vi "Close DVRs.vi"(8 "error in (no error)":errorcluster, 11 "Data":T1) -> (0 "error out":errorcluster)   [LabVIEW 2021, in "Blackboard.lvclass"]
uses:
  Blackboard.lvclass
  Blackboard.lvclass/Blackboard.ctl
  Data DVR Type.ctl
  Tags Map Type.ctl
  Data Type.ctl
  Status Type.ctl
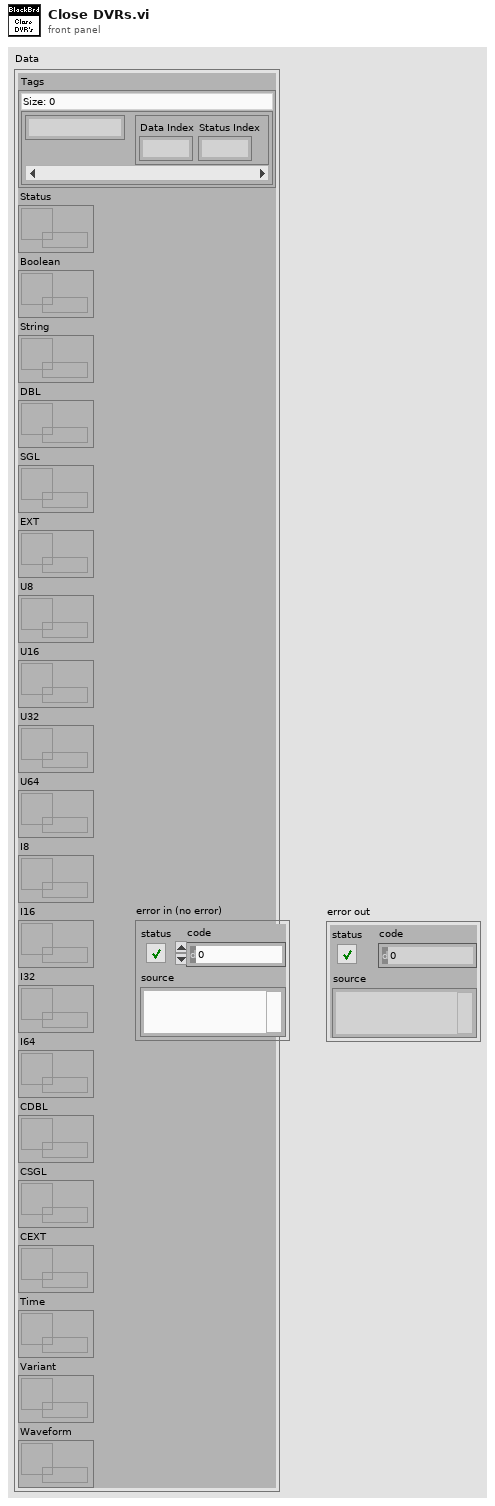
[diagram p1: front panel]
types:
  T1 = typedef "Blackboard.lvclass/Data DVR Type.ctl" = cluster{"Tags":T2, "Status":refnum<data-value>, "Boolean":refnum<data-value>, "String":refnum<data-value>, "DBL":refnum<data-value>, "SGL":refnum<data-value>, "EXT":refnum<data-value>, "U8":refnum<data-value>, "U16":refnum<data-value>, "U32":refnum<data-value>, "U64":refnum<data-value>, "I8":refnum<data-value>, "I16":refnum<data-value>, "I32":refnum<data-value>, "I64":refnum<data-value>, "CDBL":refnum<data-value>, "CSGL":refnum<data-value>, "CEXT":refnum<data-value>, "Time":refnum<data-value>, "Variant":refnum<data-value>, "Waveform":refnum<data-value>}
  T2 = typedef "Blackboard.lvclass/Tags Map Type.ctl" = map{string, cluster{"Data Index":i32, "Status Index":i32}}
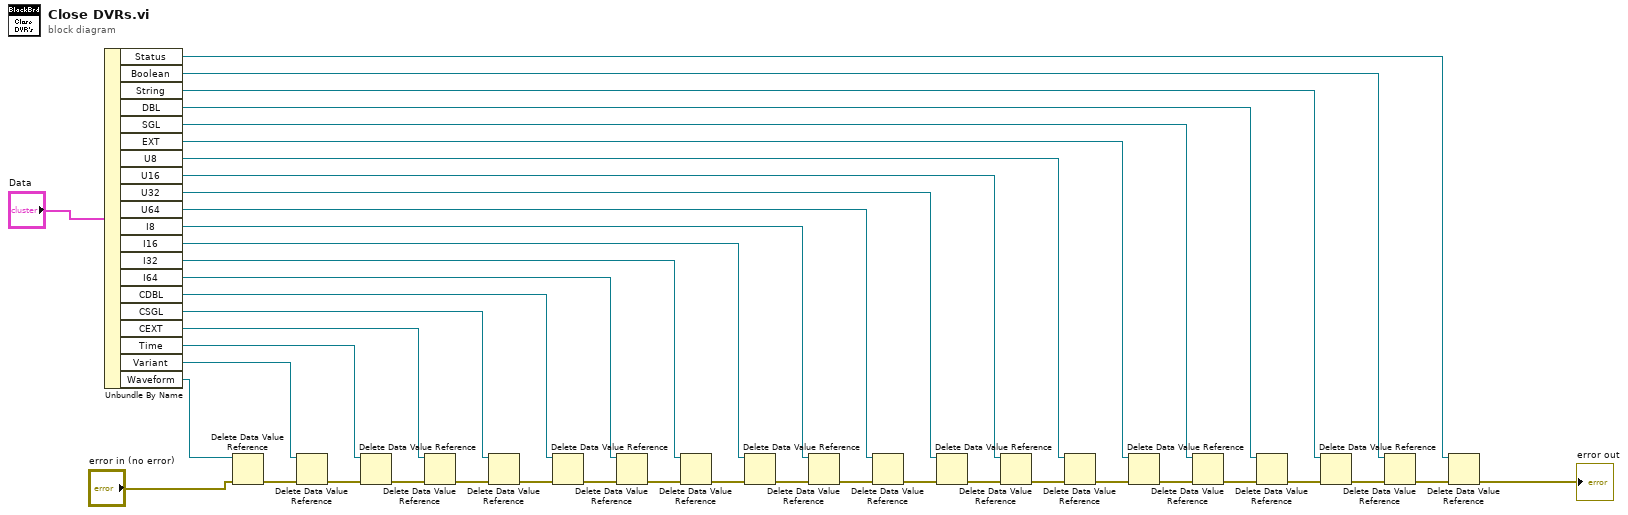
[diagram p0: block diagram]
diagram:
  n1 = Unbundle By Name("Data") -> ("Status"=w22:refnum<data-value>, "Boolean"=w23:refnum<data-value>, "String"=w24:refnum<data-value>, "DBL"=w25:refnum<data-value>, "SGL"=w26:refnum<data-value>, "EXT"=w27:refnum<data-value>, "U8"=w28:refnum<data-value>, "U16"=w29:refnum<data-value>, "U32"=w30:refnum<data-value>, "U64"=w31:refnum<data-value>, "I8"=w32:refnum<data-value>, "I16"=w33:refnum<data-value>, "I32"=w34:refnum<data-value>, "I64"=w35:refnum<data-value>, "CDBL"=w36:refnum<data-value>, "CSGL"=w37:refnum<data-value>, "CEXT"=w38:refnum<data-value>, "Time"=w39:refnum<data-value>, "Variant"=w40:refnum<data-value>, "Waveform"=w41:refnum<data-value>)
  n2 = Delete Data Value Reference(data value reference=w41, error in="error in (no error)") -> (error out=w20:errorcluster)  [unwired: 1 out]
  n3 = Delete Data Value Reference(data value reference=w40, error in=w20) -> (error out=w19:errorcluster)  [unwired: 1 out]
  n4 = Delete Data Value Reference(data value reference=w39, error in=w19) -> (error out=w18:errorcluster)  [unwired: 1 out]
  n5 = Delete Data Value Reference(data value reference=w38, error in=w18) -> (error out=w17:errorcluster)  [unwired: 1 out]
  n6 = Delete Data Value Reference(data value reference=w37, error in=w17) -> (error out=w16:errorcluster)  [unwired: 1 out]
  n7 = Delete Data Value Reference(data value reference=w36, error in=w16) -> (error out=w15:errorcluster)  [unwired: 1 out]
  n8 = Delete Data Value Reference(data value reference=w35, error in=w15) -> (error out=w14:errorcluster)  [unwired: 1 out]
  n9 = Delete Data Value Reference(data value reference=w34, error in=w14) -> (error out=w13:errorcluster)  [unwired: 1 out]
  n10 = Delete Data Value Reference(data value reference=w33, error in=w13) -> (error out=w12:errorcluster)  [unwired: 1 out]
  n11 = Delete Data Value Reference(data value reference=w32, error in=w12) -> (error out=w11:errorcluster)  [unwired: 1 out]
  n12 = Delete Data Value Reference(data value reference=w31, error in=w11) -> (error out=w10:errorcluster)  [unwired: 1 out]
  n13 = Delete Data Value Reference(data value reference=w30, error in=w10) -> (error out=w9:errorcluster)  [unwired: 1 out]
  n14 = Delete Data Value Reference(data value reference=w29, error in=w9) -> (error out=w8:errorcluster)  [unwired: 1 out]
  n15 = Delete Data Value Reference(data value reference=w28, error in=w8) -> (error out=w7:errorcluster)  [unwired: 1 out]
  n16 = Delete Data Value Reference(data value reference=w27, error in=w7) -> (error out=w6:errorcluster)  [unwired: 1 out]
  n17 = Delete Data Value Reference(data value reference=w26, error in=w6) -> (error out=w5:errorcluster)  [unwired: 1 out]
  n18 = Delete Data Value Reference(data value reference=w25, error in=w5) -> (error out=w4:errorcluster)  [unwired: 1 out]
  n19 = Delete Data Value Reference(data value reference=w24, error in=w4) -> (error out=w3:errorcluster)  [unwired: 1 out]
  n20 = Delete Data Value Reference(data value reference=w23, error in=w3) -> (error out=w2:errorcluster)  [unwired: 1 out]
  n21 = Delete Data Value Reference(data value reference=w22, error in=w2) -> (error out=→"error out":errorcluster)  [unwired: 1 out]
